vi "Pup_lower.vi"(6 "P11+dt*P31 + dt*(P13+dt*P33) + E1":fxp<+,32,16>, 9 "P13 + dt*P33 + E13":fxp<+,32,16>, 10 "output valid 32":bool, 11 "K31":fxp<+,32,16>) -> (2 "output valid 31":bool, 3 "Pup31":fxp<+,32,16>)   [LabVIEW 2020]
uses:
  <vilib>/rvi/FXPMathLib/FxpMul/XNode/nifxpmath_Multiplier.xnode
  <vilib>/rvi/FXPMathLib/FxpAdd/XNode/nifxpmath_Add.xnode
  <vilib>/rvi/FXPMathLib/sim/FxpSim.dll
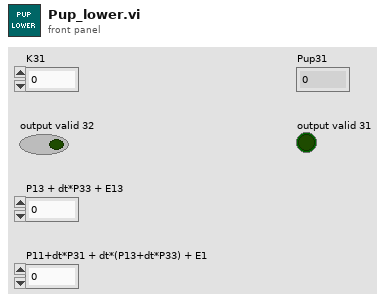
[diagram p1: front panel]
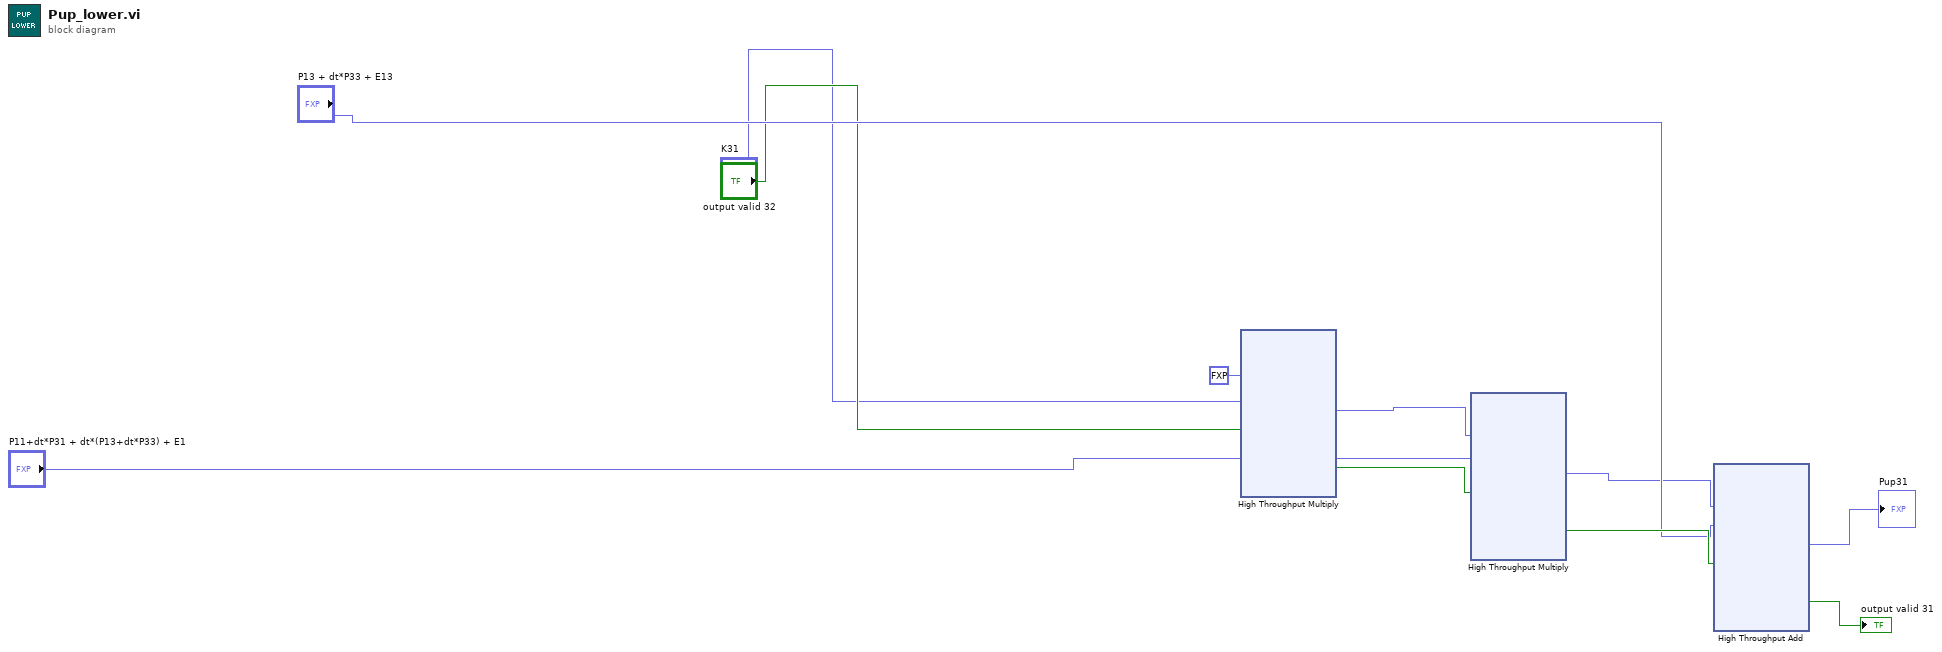
[diagram p0: block diagram]
diagram:
  n1 = xnode "High Throughput Multiply"("x"=fxp<+/-,16,1> -1.0, "y"="K31", "input valid"="output valid 32") -> ("x*y"=w4:fxp<+/-,32,16>, "output valid"=w6:bool)  [unwired: 1 in, 1 out]
  n2 = xnode "High Throughput Multiply"("x"=w4, "y"="P11+dt*P31 + dt*(P13+dt*P33) + E1", "input valid"=w6) -> ("x*y"=w7:fxp<+/-,32,16>, "output valid"=w9:bool)  [unwired: 1 in, 1 out]
  n3 = xnode "High Throughput Add"("x"=w7, "y"="P13 + dt*P33 + E13", "input valid"=w9) -> ("x+y"=→"Pup31":fxp<+,32,16>, "output valid"=→"output valid 31":bool)  [unwired: 1 in, 1 out]
